vi "Bind Property Node.vi"   [LabVIEW 2023, in "SQLite.lvlib"]
doc: "Property Node for binding values to SQL statement parameters."
uses:
  SQLite.lvlib
  SQL Statement.lvclass
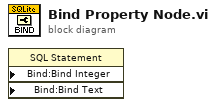
[diagram p0: block diagram]
diagram:
  n1 = property class="SQL Statement" props=["Bind:Bind Integer", "Bind:Bind Text"]() -> ()  [unwired: 4 in, 2 out]
